vi "Handle Error.vi"(8 "error in (no error)":errorcluster, 11 "SAS_AFTester_Template in":refnum<class "Business Logic Tester.lvclass">) -> (0 "error out":errorcluster, 2 "stop actor?":bool=TRUE, 3 "SAS_AFTester_Template out":refnum<class "Business Logic Tester.lvclass">)   [LabVIEW 2020, in "Business Logic Tester.lvlib" / "Business Logic Tester.lvclass"]
doc: "(<B>Filename</B>: Actor Framework.lvlib:Actor.lvclass:Handle Error.vi)\n\nDefines how the actor handles an error that occurred while processing a message. By default, this method does nothing except stop the actor."
uses:
  Business Logic Tester.lvclass
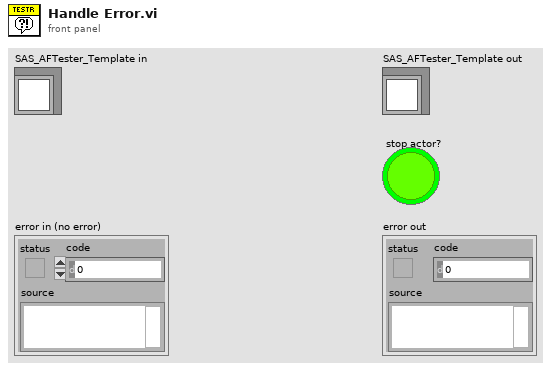
[diagram p1: front panel]
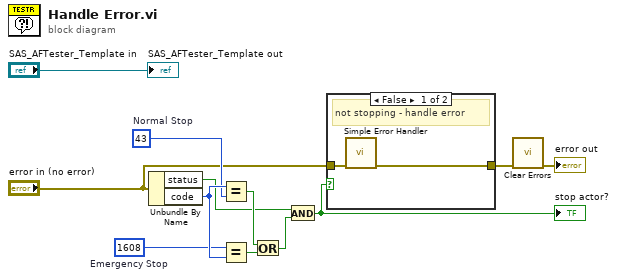
[diagram p0: block diagram]
diagram:
  w7 = 1608  # Emergency Stop
  w8 = 43  # Normal Stop
  n1 = Unbundle By Name("error in (no error)") -> ("status"=w6:bool, "code"=w9:i32)
  n2 = Equal?(x=w9, y=w8) -> (x = y?=w11:bool)
  n3 = Equal?(x=w7, y=w9) -> (x = y?=w12:bool)
  n4 = Or(x=w11, y=w12) -> (x .or. y?=w10:bool)
  n5 = And(x=w6, y=w10) -> (x .and. y?=w4:bool)
  "stop actor?" <- w4
  n6 = case shown="False" w4 {
    tunnel: "error in (no error)" -> [w14 w15]
    tunnel: [w13 w15] -> w2
    frame False {
      # "not stopping - handle error"
      n7 = call <vilib>:"Simple Error Handler.vi"("error in (no error)"=w14) -> ("error out"=w13:errorcluster)  [unwired: 4 in, 4 out]
    }
    frame True {
      # "Stopping - Do nothing"
    }
  }
  n8 = call <vilib>:"Clear Errors.vi"("error in (no error)"=w2) -> ("error out"=→"error out":errorcluster)  [unwired: 5 in, 1 out]
  "SAS_AFTester_Template out" <- "SAS_AFTester_Template in"
